vi "Global.vi"() -> ()   [LabVIEW 2011]
panel:
  out "Effective field [T]":dbl[unit] format="%.3f"
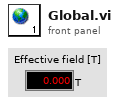
[diagram p1: front panel]
diagram:
